vi "V2 To V3 Upgrade Refactory Data.vi"() -> (0 "refactor data":T1)   [LabVIEW 2020, in "MeasurementService Editor.lvlib"]
uses:
  MeasurementService Editor.lvlib
  Rename Refactor Data.ctl
  Rename Refactor Mapping Info.ctl
  Rename String Mapping.ctl
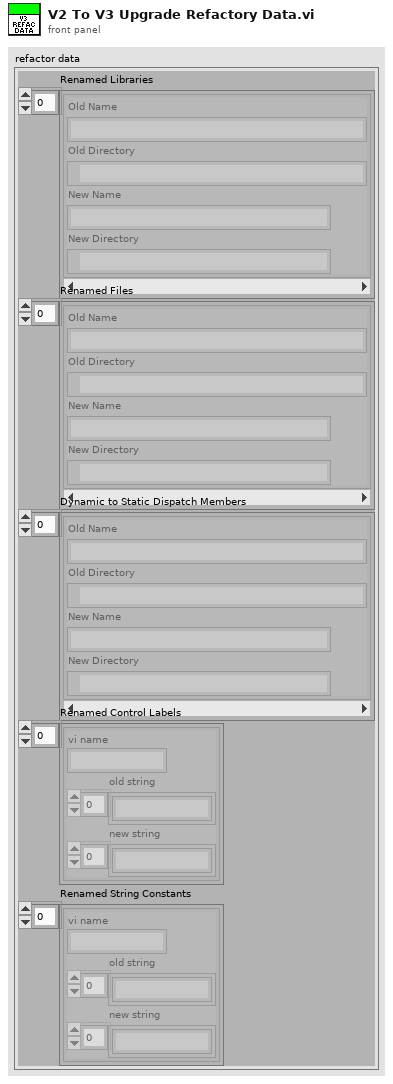
[diagram p1: front panel]
types:
  T1 = typedef "MeasurementService Editor.lvlib/Rename Refactor Data.ctl" = cluster{"Renamed Libraries":T2[], "Renamed Files":T2[], "Dynamic to Static Dispatch Members":T2[], "Renamed Control Labels":T3[], "Renamed String Constants":T3[]}
  T2 = typedef "MeasurementService Editor.lvlib/Rename Refactor Mapping Info.ctl" = cluster{"Old Name":string, "Old Directory":path, "New Name":string, "New Directory":path}
  T3 = typedef "MeasurementService Editor.lvlib/Rename String Mapping.ctl" = cluster{"vi name":string, "old string":string[], "new string":string[]}
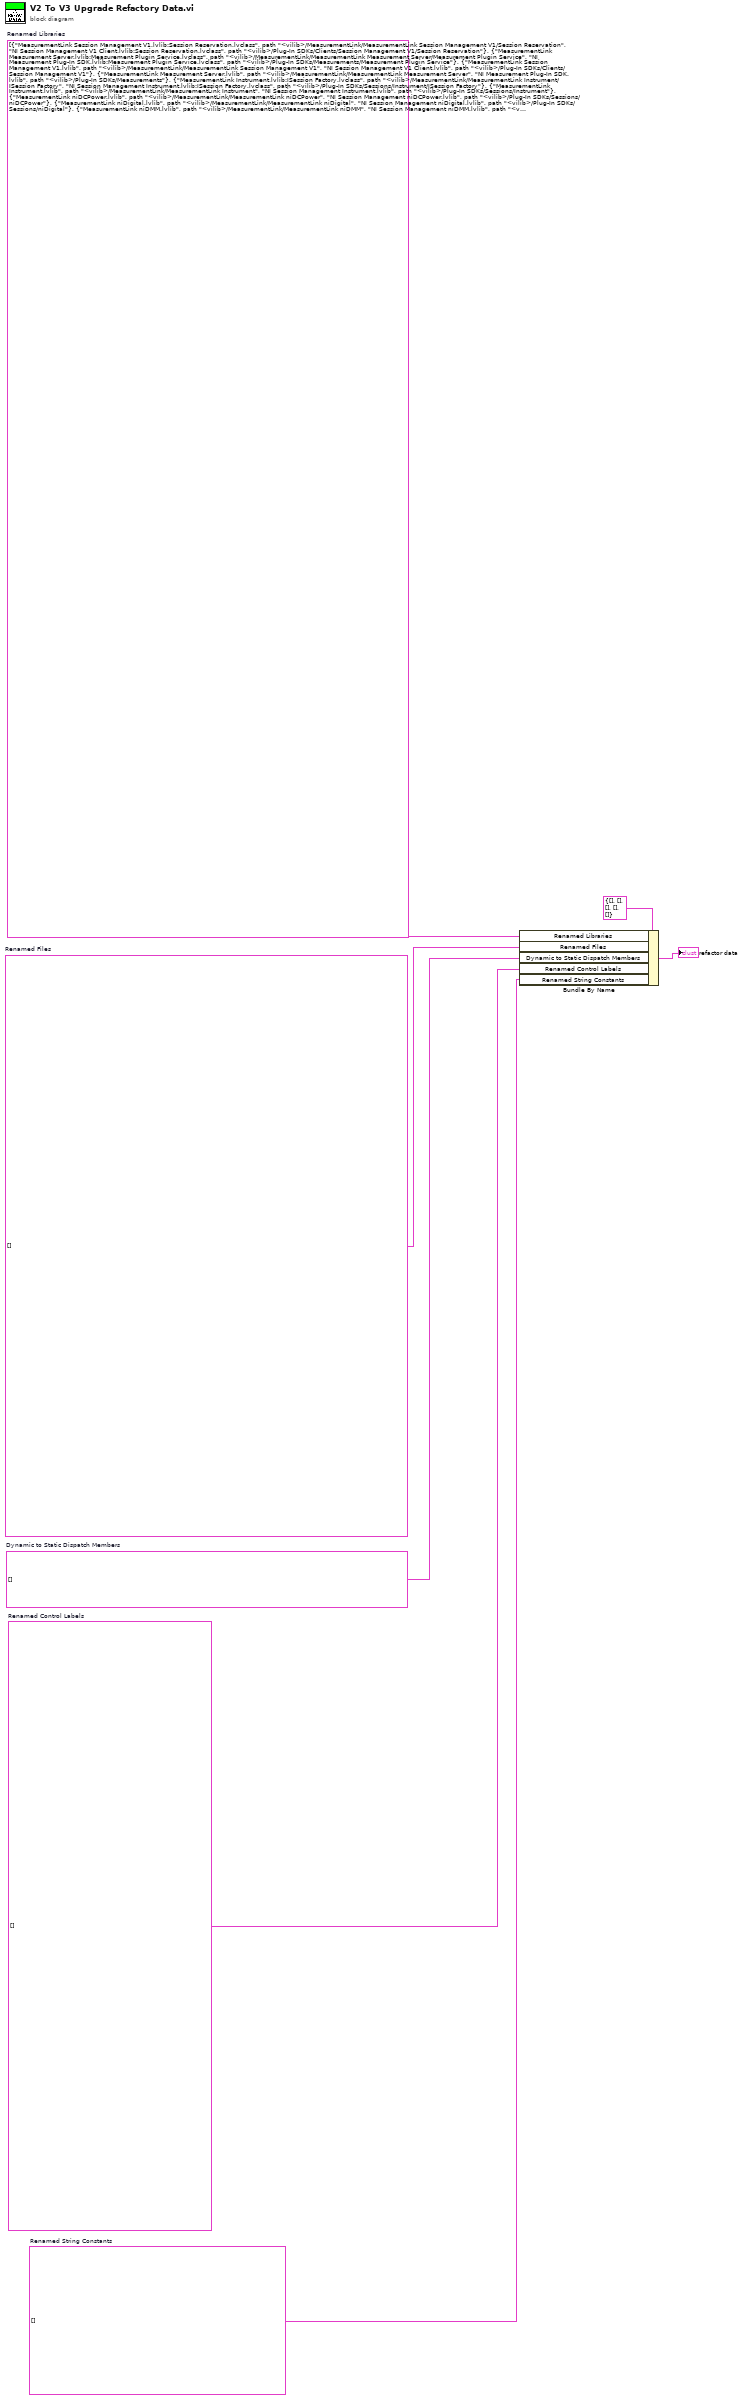
[diagram p0: block diagram]
diagram:
  w1 = T3[] []  # Renamed String Constants
  w2 = T3[] []  # Renamed Control Labels
  w3 = T2[] []  # Dynamic to Static Dispatch Members
  w4 = T2[] []  # Renamed Files
  w6 = T2[] [{"Old Name"="MeasurementLink Session Management V1.lvlib:Session Reservation.lvclass", "Old Directory"=path "<vilib>/MeasurementLink/MeasurementLink Session Management V1/Session Reservation", "New Name"="NI Session Management V1 Client.lvlib:Session Reservation.lvclass", "New Directory"=path "<vilib>/Plug-In SDKs/Clients/Session Management V1/Session Reservation"}, {"Old Name"="MeasurementLink Measurement Server.lvlib:Measurement Plugin Service.lvclass", "Old Directory"=path "<vilib>/MeasurementLink/MeasurementLink Measurement Server/Measurement Plugin Service", "New Name"="NI Measurement Plug-In SDK.lvlib:Measurement Plugin Service.lvclass", "New Directory"=path "<vilib>/Plug-In SDKs/Measurements/Measurement Plugin Service"}, {"Old Name"="MeasurementLink Session Management V1.lvlib", "Old Directory"=path "<vilib>/MeasurementLink/MeasurementLink Session Management V1", "New Name"="NI Session Management V1 Client.lvlib", "New Directory"=path "<vilib>/Plug-In SDKs/Clients/Session Management V1"}, {"Old Name"="MeasurementLink Measurement Server.lvlib", "Old Directory"=path "<vilib>/MeasurementLink/MeasurementLink Measurement Server", "New Name"="NI Measurement Plug-In SDK.lvlib", "New Directory"=path "<vilib>/Plug-In SDKs/Measurements"}, {"Old Name"="MeasurementLink Instrument.lvlib:ISession Factory.lvclass", "Old Directory"=path "<vilib>/MeasurementLink/MeasurementLink Instrument/ISession Factory", "New Name"="NI Session Management Instrument.lvlib:ISession Factory.lvclass", "New Directory"=path "<vilib>/Plug-In SDKs/Sessions/Instrument/ISession Factory"}, {"Old Name"="MeasurementLink Instrument.lvlib", "Old Directory"=path "<vilib>/MeasurementLink/MeasurementLink Instrument", "New Name"="NI Session Management Instrument.lvlib", "New Directory"=path "<vilib>/Plug-In SDKs/Sessions/Instrument"}, {"Old Name"="MeasurementLink niDCPower.lvlib", "Old Directory"=path "<vilib>/MeasurementLink/MeasurementLink niDCPower", "New Name"="NI Session Management niDCPower.lvlib", "New Directory"=path "<vilib>/Plug-In SDKs/Sessions/niDCPower"}, {"Old Name"="MeasurementLink niDigital.lvlib", "Old Directory"=path "<vilib>/MeasurementLink/MeasurementLink niDigital", "New Name"="NI Session Management niDigital.lvlib", "New Directory"=path "<vilib>/Plug-In SDKs/Sessions/niDigital"}, {"Old Name"="MeasurementLink niDMM.lvlib", "Old Directory"=path "<vilib>/MeasurementLink/MeasurementLink niDMM", "New Name"="NI Session Management niDMM.lvlib", "New Directory"=path "<vilib>/Plug-In SDKs/Sessions/niDMM"}, {"Old Name"="MeasurementLink niFGEN.lvlib", "Old Directory"=path "<vilib>/MeasurementLink/MeasurementLink niFGEN", "New Name"="NI Session Management niFGEN.lvlib", "New Directory"=path "<vilib>/Plug-In SDKs/Sessions/niFGEN"}, {"Old Name"="MeasurementLink niScope.lvlib", "Old Directory"=path "<vilib>/MeasurementLink/MeasurementLink niScope", "New Name"="NI Session Management niScope.lvlib", "New Directory"=path "<vilib>/Plug-In SDKs/Sessions/niScope"}, {"Old Name"="MeasurementLink VISA.lvlib", "Old Directory"=path "<vilib>/MeasurementLink/MeasurementLink VISA", "New Name"="NI Session Management VISA.lvlib", "New Directory"=path "<vilib>/Plug-In SDKs/Sessions/VISA"}, {"Old Name"="MeasurementLink Measurement Server Internal.lvlib", "Old Directory"=path "<vilib>/MeasurementLink/MeasurementLink Measurement Server Internal", "New Name"="ni.measurementlink.measurement.v1.api.lvlib", "New Directory"=path "<vilib>/gRPC/Generated APIs/ni/measurementlink/measurement/v1"}, {"Old Name"="MeasurementLink Measurement Service Base V2.lvlib", "Old Directory"=path "<vilib>/MeasurementLink/MeasurementLink Measurement Service Base V2", "New Name"="ni.measurementlink.measurement.v2.api.lvlib", "New Directory"=path "<vilib>/gRPC/Generated APIs/ni/measurementlink/measurement/v2"}, {"Old Name"="MeasurementLink TestStand Integration.lvlib", "Old Directory"=path "<vilib>/MeasurementLink/MeasurementLink TestStand Integration", "New Name"="NI Pin Map TestStand.lvlib", "New Directory"=path "<vilib>/Plug-In SDKs/TestStand"}]  # Renamed Libraries
  n1 = Bundle By Name(cluster=T1 {"Renamed Libraries"=[], "Renamed Files"=[], "Dynamic to Static Dispatch Members"=[], "Renamed Control Labels"=[], "Renamed String Constants"=[]} ("Rename Data"), "Renamed Libraries"=w6, "Renamed Files"=w4, "Dynamic to Static Dispatch Members"=w3, "Renamed Control Labels"=w2, "Renamed String Constants"=w1) -> (→"refactor data":T1)
